vi "Table, Set Color.vi"(4 "Enable (T)":bool=TRUE, 5 "BGColor Default":u32(colorbox)=16448250, 6 "BGColor Enabled":u32(colorbox)=16777215, 7 "error in":errorcluster, 10 "Tbl Refnum":refnum<vi>) -> (0 "error out":errorcluster, 3 "Tbl Refnum out":refnum<vi>)   [LabVIEW 2010]
doc: "Sets the active table cell and changes its background color attribute."
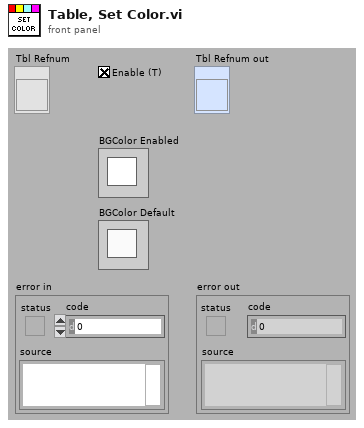
[diagram p1: front panel]
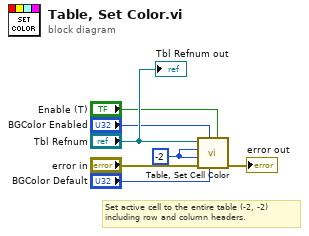
[diagram p0: block diagram]
diagram:
  w5 = -2 ("row (0)")
  # "Set active cell to the entire table (-2, -2)\nincluding row and column headers."
  n1 = call "Table, Set Cell Color.vi"("Enable (T)"="Enable (T)", "BGColor Default"="BGColor Default", "BGColor Enabled"="BGColor Enabled", "error in"="error in", "col (0)"=w5, "row (0)"=w5, "Tbl Refnum"="Tbl Refnum") -> ("error out"=→"error out":errorcluster)  [unwired: 3 out]
  "Tbl Refnum out" <- "Tbl Refnum"
